vi "readMsg TEST.vi"() -> ()   [LabVIEW 2019]
uses:
  <vilib>/rvi/Emulation/niFpgaGetClockAttributes.vi
  <vilib>/rvi/Emulation/niFpgaSctlEmulationGetInTimedLoop.vi
  <vilib>/rvi/Emulation/niFpgaEmulationReportErrorSimple.vi
  <vilib>/rvi/Emulation/niFpgaProcessEmulError.vi
  <vilib>/rvi/Emulation/niFpgaCriticalErrorInLSC.vi
panel:
  out "Read Data?":bool
  in  "stop":bool
  out "CAN Msg":u8[](array[numeric]) format="%02x"
  out "ID":u32 format="%x"
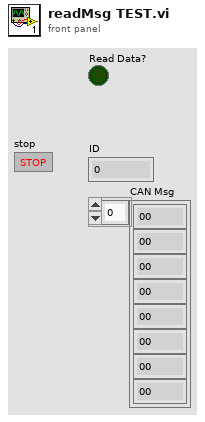
[diagram p1: front panel]
types:
  T1 = enum16{"100kBPS", "250kBPS", "500kBPS", "1000kBPS"}
  T2 = typedef "SPI Config.ctl" = cluster{"MXP Port":enum16{"A", "B"}, "Device":enum16{"CAN", "ENC", "IMU1", "IMU2"}, "CPOL":bool}
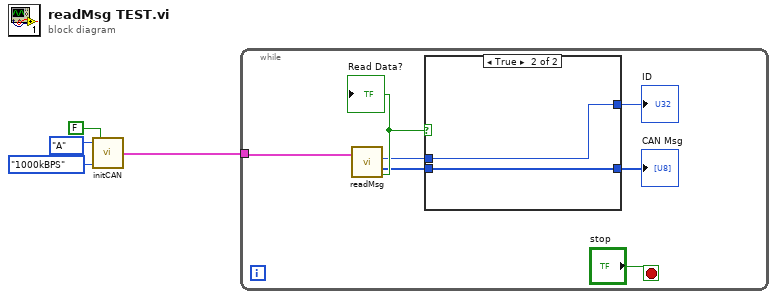
[diagram p0: block diagram]
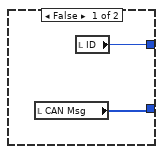
[diagram p2: hidden frame]
diagram:
  n1 = call "initCAN.vi"("Baud Rate"=T1."1000kBPS", "CPOL"=FALSE, "MXP Port"=enum16{"A", "B"}."A") -> ("SPI Config Out"=w4:T2)
  n2 = while {
    tunnel: w4 -> [w11]
    stop <- "stop" stop-if-true
    n3 = call "readMsg.vi"("SPI Config In"=w11) -> ("ID"=w7:u32, "CAN Msg"=w5:u8[], "Read Data?"=w9:bool)  [unwired: 1 in, 1 out]
    "Read Data?" <- w9
    n4 = case shown="True" w9 {
      tunnel: [w12 w15] -> w8
      tunnel: w7 -> [_ w15]
      tunnel: [w13 w14] -> w6
      tunnel: w5 -> [_ w14]
      frame False {
        n5 = local read "CAN Msg"() -> (w13:u8[])
        n6 = local read "ID"() -> (w12:u32)
      }
      frame True {
      }
    }
    "ID" <- w8
    "CAN Msg" <- w6
  }
